vi "IV(H)_DC_vector_magnetsweep_BF_LD-400_K6221_K2182A_PK.vi"() -> ()   [LabVIEW 2016]
uses:
  LabView_Switching exp/SubVI/Keithley 622x LV 8.0/Keithley 622x.lvlib
panel:
  in  "Set Compliance voltage (V)":dbl=2.0 min=0.0 step=0.1 format="%_3f"
  in  "Step 3":dbl[](array[numeric])=[1e-07, 1e-07, 1e-07, 1e-07, 1e-07] min=-3000.0 max=3000.0 format="%.1e"
  in  "To 3":dbl[](array[numeric])=[2e-05, -2e-05, 2e-05, -2e-05, 0.0] min=-3000.0 max=3000.0 format="%.1e"
  in  "From 3":dbl[](array[numeric])=[0.0, 2e-05, -2e-05, 2e-05, -2e-05] min=-3000.0 max=3000.0 format="%.1e"
  in  "wait (ms)":u32=1000
  in  "Nanovoltmeter 2182a VISA":refnum<visa-resource-name>="GPIB0::4::INSTR"
  in  "Current source K6221 VISA":refnum<visa-resource-name>="GPIB0::12::INSTR"
  in  "Number Averaging":i32=50
  in  "Tab Control":enum32{"Page 1", "Page 2"}(tab)
  out "V vs I":cluster{dbl, "Field Reading":dbl}[](graph)=[{88.00020049365409, "Field Reading"=1178949.0151954973}, {88.04984142978704, "Field Reading"=1177290.5042515406}, {88.09983377178898, "Field Reading"=1169991.8797237715}, {88.14983820874596, "Field Reading"=1131113.310921174}, {88.1998015211176, "Field Reading"=1135549.0095311047}, {88.24974082906098, "Field Reading"=1140239.9000253335}, {88.29974217872491, "Field Reading"=1145253.1684029822}, {88.34980121180439, "Field Reading"=1125822.473165846}, {88.39976089537811, "Field Reading"=1100990.7144727584}, {88.44976462735649, "Field Reading"=1124277.980977591}, {88.49991354243424, "Field Reading"=1113133.7403579995}, {88.549835629691, "Field Reading"=1095078.3421750271}, {88.59973785169807, "Field Reading"=1089005.9296407204}, {88.64981796279662, "Field Reading"=1071016.6334025378}, {88.69999071622563, "Field Reading"=1068470.5118392052}, {88.74987372198214, "Field Reading"=1063537.6502689242}, {88.79982875283143, "Field Reading"=1037928.4122448568}, {88.84986306680204, "Field Reading"=1023763.2014216684}, {88.89976547995889, "Field Reading"=1020228.703507441}, {88.94984930717325, "Field Reading"=1000335.3237807469}, {88.99981793410211, "Field Reading"=965050.429505623}, {89.04974778345694, "Field Reading"=978646.5702332633}, {89.09972081248361, "Field Reading"=961519.051741358}, {89.14993565961254, "Field Reading"=939591.945473506}, {89.199725161219, "Field Reading"=918130.4335429888}, {89.24992589877172, "Field Reading"=906781.4220801867}, {89.29974686814681, "Field Reading"=861156.5000297616}, {89.34974265040302, "Field Reading"=831340.4861009503}, {89.39976422439847, "Field Reading"=827959.2552652409}, {89.44974554488792, "Field Reading"=794041.0257164304}, {89.49998047914683, "Field Reading"=792136.3577627148}, {89.54988391763179, "Field Reading"=826457.2883509871}, {89.59982657379398, "Field Reading"=877464.375741542}, {89.64995889945494, "Field Reading"=903593.98825095}, {89.69977125493678, "Field Reading"=917153.966335848}, {89.75002893453679, "Field Reading"=947464.6903531018}, {89.79975720608076, "Field Reading"=968432.2031485286}, {89.84972844020538, "Field Reading"=977841.59734809}, {89.89977155512094, "Field Reading"=992923.8733686475}, {89.9498829635706, "Field Reading"=1004882.2444193498}, {89.99973795869549, "Field Reading"=1028335.1131184339}, {90.04983989122205, "Field Reading"=1025131.272606909}, {90.09994908920751, "Field Reading"=1041173.1024543894}, {90.14982036437434, "Field Reading"=1059237.6751508159}, {90.19980108193258, "Field Reading"=1067565.6836621398}, {90.24973246359373, "Field Reading"=1080472.0318337064}, {90.29996005213907, "Field Reading"=1088475.3372523}, {90.34983233834966, "Field Reading"=1097983.7020025607}, {90.39974610255554, "Field Reading"=1110923.2678247455}, {90.44980343772909, "Field Reading"=1137279.5384549182}, {90.49985241598829, "Field Reading"=1133355.3807623477}, {90.54979294346053, "Field Reading"=1161334.2887808664}, {90.59979410780464, "Field Reading"=1162461.6397829298}, {90.64974434482343, "Field Reading"=1154218.0501570704}, {90.69986742044274, "Field Reading"=1175023.037400592}, {90.74975392715889, "Field Reading"=1158309.8392327735}, {90.80003104609368, "Field Reading"=1160751.9247400747}, {90.84999133832466, "Field Reading"=1180373.5089674825}, {90.89971363302666, "Field Reading"=1178207.0893623114}, {90.9498700750375, "Field Reading"=1186215.801522418}, {90.99972893957116, "Field Reading"=1201413.7681875122}, {91.04977648059084, "Field Reading"=1208681.2076781155}, {91.09985585712178, "Field Reading"=1197895.0972802779}, {91.14982332628642, "Field Reading"=1210652.407715155}, {91.19971838168068, "Field Reading"=1230701.8068384205}, {91.24976729118956, "Field Reading"=1223512.0994189004}, {91.2998516329973, "Field Reading"=1211497.4848096254}, {91.35001158581667, "Field Reading"=1236879.1492508247}, {91.39973785948087, "Field Reading"=1225471.6410425988}, {91.44993058632726, "Field Reading"=1213253.058893187}, {91.49972258715553, "Field Reading"=1210915.25397176}, {91.54988360100296, "Field Reading"=1209863.3661352952}, {91.60003041097399, "Field Reading"=1221964.611924381}, {91.64973262548213, "Field Reading"=1219022.0454230926}, {91.69978400884942, "Field Reading"=1235046.803652391}, {91.74994445658069, "Field Reading"=1232760.0066260807}, {91.80022524347947, "Field Reading"=1256153.8474325093}, {91.8497947448095, "Field Reading"=1241071.9759753507}, {91.89977761295827, "Field Reading"=1249134.9364484414}, {91.94975866856626, "Field Reading"=1235919.8359682774}, {91.99996795172356, "Field Reading"=1235542.8724599753}]
  out "V vs time":cluster{dbl, "Field Reading":dbl}[](graph)=[{1.9999967297364587, "Field Reading"=1178949.0151954973}, {1.999994153904603, "Field Reading"=1177290.5042515406}, {1.9999989129086975, "Field Reading"=1169991.8797237715}, {1.9999918946491422, "Field Reading"=1131113.310921174}, {2.0000099968351024, "Field Reading"=1135549.0095311047}, {1.9999924050786144, "Field Reading"=1140239.9000253335}, {2.0000036443721094, "Field Reading"=1145253.1684029822}, {1.9999972262759285, "Field Reading"=1125822.473165846}, {2.000007931072924, "Field Reading"=1100990.7144727584}, {2.0000066284007425, "Field Reading"=1124277.980977591}, {1.9999952434214299, "Field Reading"=1113133.7403579995}, {1.999996661070107, "Field Reading"=1095078.3421750271}, {2.000006659018672, "Field Reading"=1089005.9296407204}, {2.0000039383733044, "Field Reading"=1071016.6334025378}, {2.0000048869646743, "Field Reading"=1068470.5118392052}, {2.000005777378757, "Field Reading"=1063537.6502689242}, {2.0000049123234382, "Field Reading"=1037928.4122448568}, {1.9999948449122227, "Field Reading"=1023763.2014216684}, {1.9999942408675742, "Field Reading"=1020228.703507441}, {1.999997049209919, "Field Reading"=1000335.3237807469}, {1.9999992434973093, "Field Reading"=965050.429505623}, {2.0000055966816648, "Field Reading"=978646.5702332633}, {1.99999211416235, "Field Reading"=961519.051741358}, {1.999997937140985, "Field Reading"=939591.945473506}, {1.9999920221749543, "Field Reading"=918130.4335429888}, {2.0000099655654218, "Field Reading"=906781.4220801867}, {1.9999941922138977, "Field Reading"=861156.5000297616}, {2.000001391498262, "Field Reading"=831340.4861009503}, {2.000008695947139, "Field Reading"=827959.2552652409}, {1.9999970142052288, "Field Reading"=794041.0257164304}, {2.000004081973531, "Field Reading"=792136.3577627148}, {1.999992656312225, "Field Reading"=826457.2883509871}, {2.0000052739895784, "Field Reading"=877464.375741542}, {2.0000002562870884, "Field Reading"=903593.98825095}, {2.000001858354245, "Field Reading"=917153.966335848}, {1.9999982641352978, "Field Reading"=947464.6903531018}, {1.9999988882792294, "Field Reading"=968432.2031485286}, {2.0000003937283735, "Field Reading"=977841.59734809}, {2.000000600107891, "Field Reading"=992923.8733686475}, {2.000000719113082, "Field Reading"=1004882.2444193498}, {2.000007198020917, "Field Reading"=1028335.1131184339}, {1.9999974916731693, "Field Reading"=1025131.272606909}, {2.0000048080798685, "Field Reading"=1041173.1024543894}, {1.9999906954500268, "Field Reading"=1059237.6751508159}, {1.9999915914078321, "Field Reading"=1067565.6836621398}, {2.0000082879110646, "Field Reading"=1080472.0318337064}, {1.9999953701409292, "Field Reading"=1088475.3372523}, {1.9999996077684985, "Field Reading"=1097983.7020025607}, {2.0000055728717165, "Field Reading"=1110923.2678247455}, {1.9999980037725664, "Field Reading"=1137279.5384549182}, {1.999996384784627, "Field Reading"=1133355.3807623477}, {2.000004103884631, "Field Reading"=1161334.2887808664}, {1.999993443662003, "Field Reading"=1162461.6397829298}, {2.0000021944025916, "Field Reading"=1154218.0501570704}, {1.99999483275991, "Field Reading"=1175023.037400592}, {1.999992715812885, "Field Reading"=1158309.8392327735}, {2.000008000892638, "Field Reading"=1160751.9247400747}, {2.0000043390415403, "Field Reading"=1180373.5089674825}, {2.000008103048867, "Field Reading"=1178207.0893623114}, {1.999990483426892, "Field Reading"=1186215.801522418}, {1.9999901120733596, "Field Reading"=1201413.7681875122}, {1.9999899676610864, "Field Reading"=1208681.2076781155}, {2.000002438619714, "Field Reading"=1197895.0972802779}, {1.99999522928944, "Field Reading"=1210652.407715155}, {2.0000031718988076, "Field Reading"=1230701.8068384205}, {1.9999936301375478, "Field Reading"=1223512.0994189004}, {2.0000077808662033, "Field Reading"=1211497.4848096254}, {2.000008829542967, "Field Reading"=1236879.1492508247}, {2.0000094317080235, "Field Reading"=1225471.6410425988}, {1.9999968576261167, "Field Reading"=1213253.058893187}, {2.000006785911426, "Field Reading"=1210915.25397176}, {1.9999948229255613, "Field Reading"=1209863.3661352952}, {2.000000480747043, "Field Reading"=1221964.611924381}, {2.0000096398922595, "Field Reading"=1219022.0454230926}, {2.0000067770884993, "Field Reading"=1235046.803652391}, {1.9999916662317956, "Field Reading"=1232760.0066260807}, {1.9999971428402814, "Field Reading"=1256153.8474325093}, {1.9999922852387555, "Field Reading"=1241071.9759753507}, {1.9999900072628842, "Field Reading"=1249134.9364484414}, {2.000006765222829, "Field Reading"=1235919.8359682774}, {2.0000011636290265, "Field Reading"=1235542.8724599753}]
  out "Magnetic Field Vector Angle":dbl=91.99996795172356 format="%#_13g"
  out "Magnetic Field Vector magnitude (T)":dbl=2.0000011636290265 format="%#_13g"
  in  "From 2":dbl[](array[numeric])=[2.0] min=-3000.0 max=3000.0 format="%.1g"
  in  "To 2":dbl[](array[numeric])=[2.0] min=-3000.0 max=3000.0 format="%.1g"
  in  "Step 2":dbl[](array[numeric])=[0.5] min=-3000.0 max=3000.0 format="%.3g"
  in  "Wait time after each sweep(min)":dbl=10.0 format="%#_13g"
  out "Z-axis Magnetic Field (T)":string="1.998782856\r\n"
  in  "Y-axis Field ramp rate (T/min)":string="0.01"
  in  "Z-axis Field ramp rate (T/min)":string="0.05"
  out "Z-axis":dbl(slide)=1.998782856 scale=0.0..3.0
  out "Y-Axis":dbl(slide)=-0.069797916 scale=0.0..3.0
  out "Y-axis Magnetic Field (T)":string="-0.069797916\r\n"
  in  "Magnet IP Address Z-axis":string="169.254.239.127"
  in  "Magnet IP Address Y-axis":string="169.254.109.232"
  out "Resistance (ohm)":dbl=1235542.8724599753 format="%#_13g"
  out "Time (s)":dbl=3083.965 format="%#_13g"
  in  "Magnetic field stabilization time (s)":dbl=10.0 format="%#_13g"
  in  "Step":dbl[](array[numeric])=[0.05] min=-3000.0 max=3000.0 format="%.3g"
  in  "To":dbl[](array[numeric])=[92.0] min=-3000.0 max=3000.0 format="%.1f"
  in  "From":dbl[](array[numeric])=[88.0] min=-3000.0 max=3000.0 format="%.1f"
  out "Iset (A)":dbl=3.2552506860087776e-11
  out "Vmeas (V)":dbl=4.02200178316859e-05
  in  "Folder":path=path "D:/Pranava/Data/STS/MA2158 new mask"
  out "data":dbl[](array[numeric])=[2.0000011636290265, 91.99996795172356, 4.02200178316859e-05, 3.2552506860087776e-11, 1235542.8724599753, 3083.965]
  in  "File name":string="009_MA2158[Dev90]_R(A)_baseT_stable_2T_vector_40uV_50ave"
  out "File path":path=path "D:/Pranava/Data/STS/MA2158 new mask/009_MA2158[Dev90]_R(A)_baseT_stable_2T_vector_40uV_50ave.dat"
  # "Z-Axis: In-plane (90 deg)\nY-axis: Out-of-plane (0 deg)"
  # "[Must be less than 0.05]"
  # ".dat"
  # "It is important that there is enough time for the magnet to cool down after each sweep (Typically 15-20 min)"
  # "Configure Field magnitude (T)"
  # "Configure Field Angle (deg)"
  # "Configure current sweeps (A)"
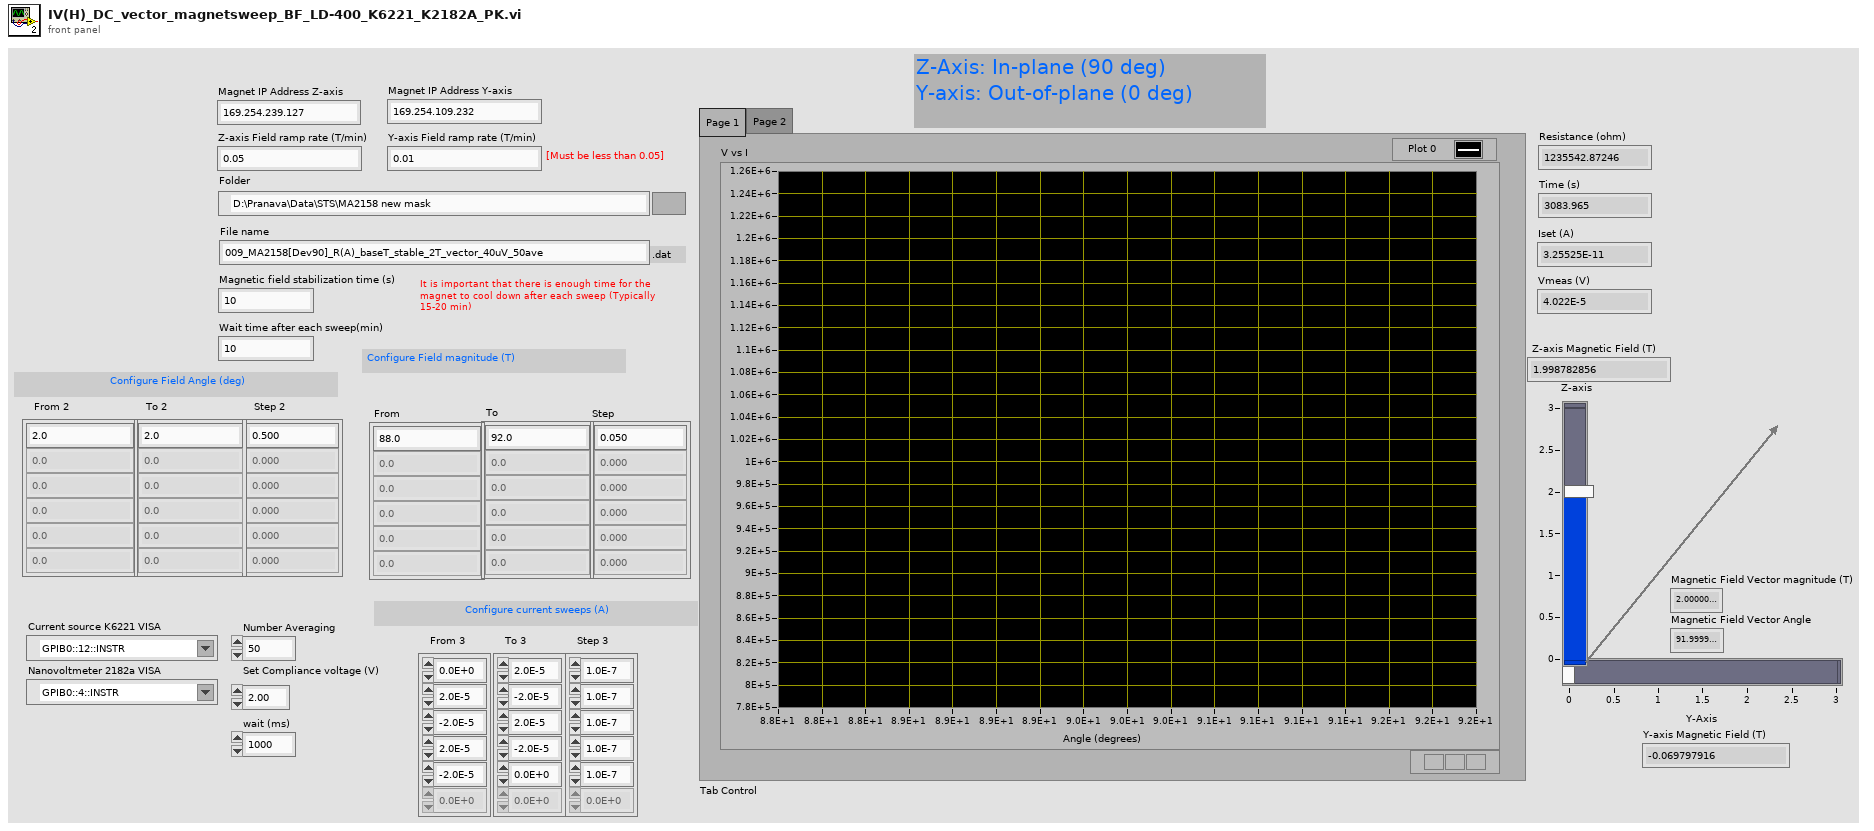
[diagram p1: front panel]
types:
  T1 = enum16{"open", "replace", "create", "open or create", "replace or create", "replace or create with confirmation"}
  T2 = typedef "Keithley 622x.lvlib/KE622x -- Current Level.ctl" = dbl
  T3 = cluster{"Current Level (A)":T2, "Field Reading":dbl}[]
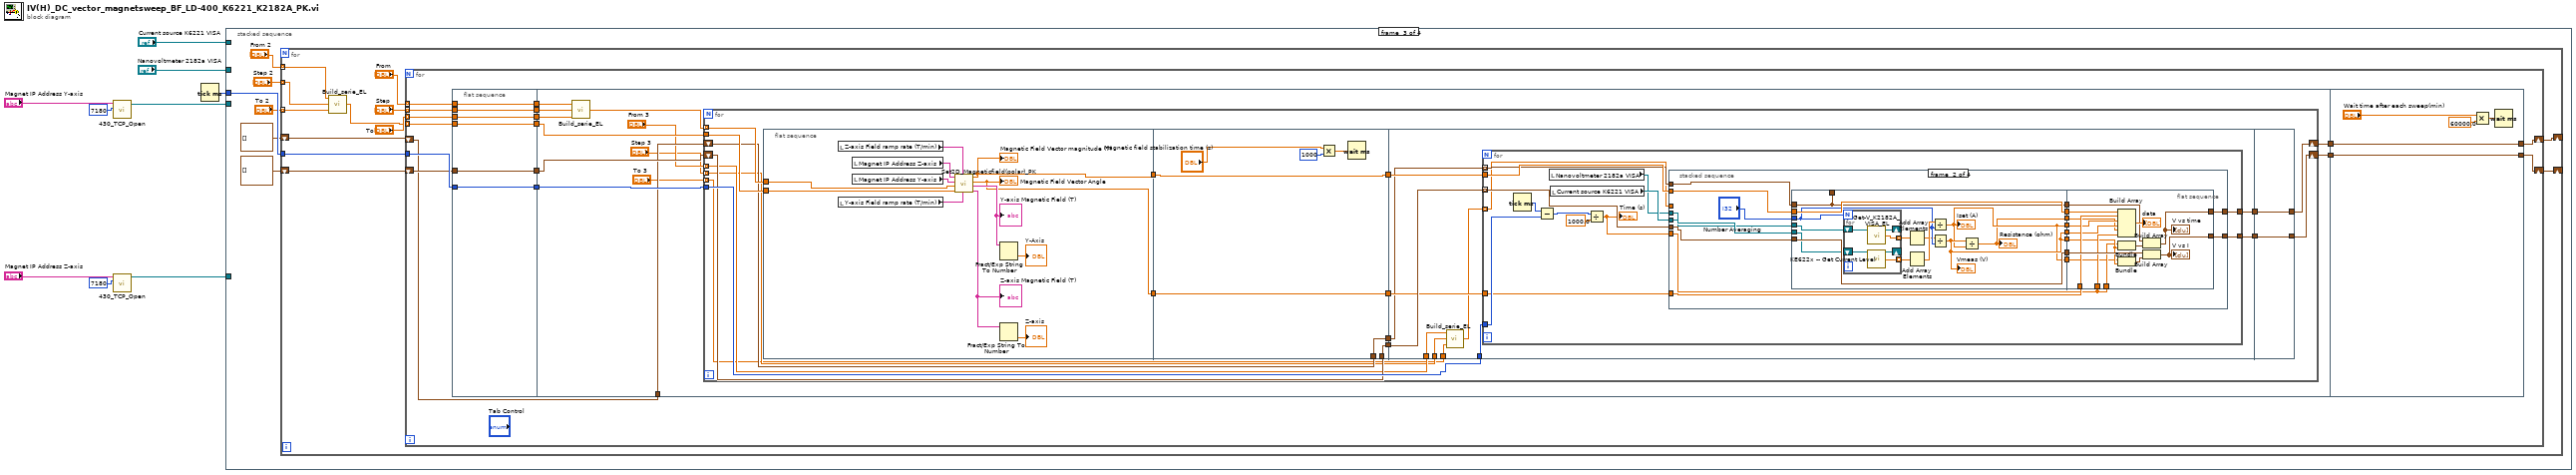
[diagram p0: block diagram]
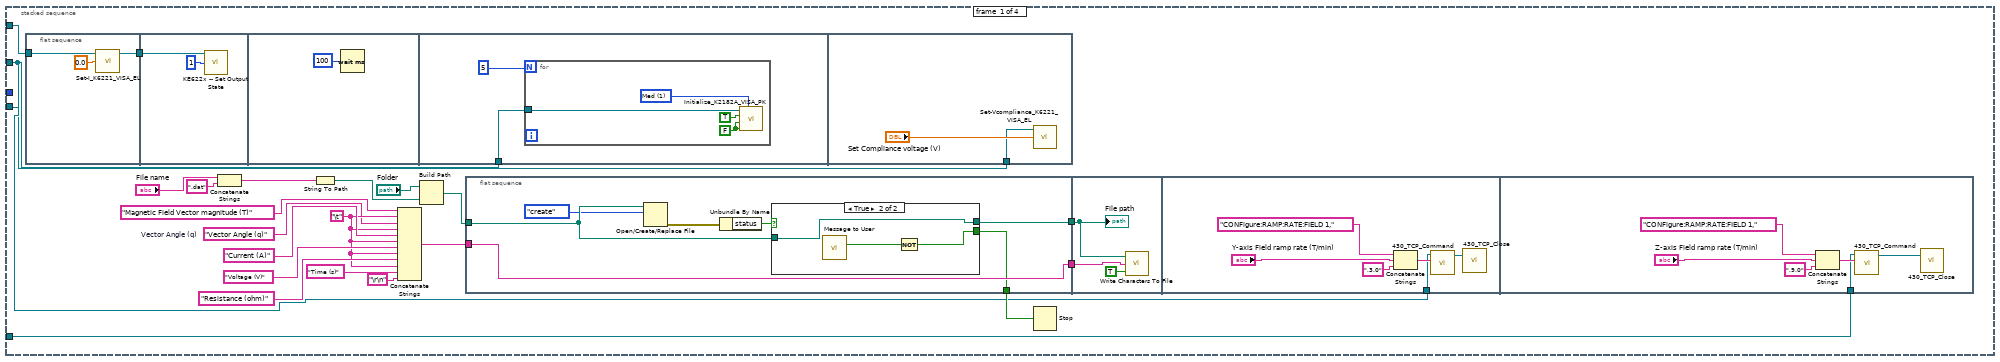
[diagram p2: hidden frame]
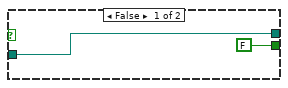
[diagram p3: hidden frame]
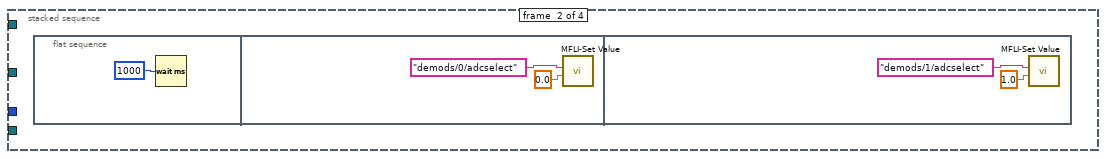
[diagram p4: hidden frame]
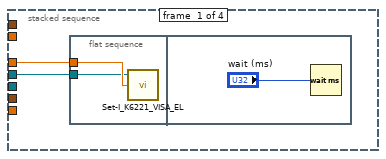
[diagram p5: hidden frame]
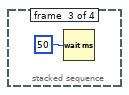
[diagram p6: hidden frame]
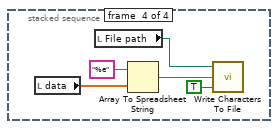
[diagram p7: hidden frame]
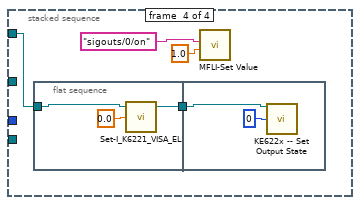
[diagram p8: hidden frame]
diagram:
  n1 = call "430_TCP_Open.vi"("IP Address"="Magnet IP Address Y-axis", "TCP Port"=7180) -> ("connection ID"=w8:refnum<k5>)  [unwired: 4 in, 2 out]
  n2 = call "430_TCP_Open.vi"("IP Address"="Magnet IP Address Z-axis", "TCP Port"=7180) -> ("connection ID"=w3:refnum<k5>)  [unwired: 4 in, 2 out]
  n3 = Tick Count (ms)() -> (millisecond timer value=w7:u32)
  n4 = stacked-sequence {
    tunnel: w8 -> [w18 _ _ _]
    tunnel: w7 -> [_ _ w84 _]
    tunnel: w3 -> [w15 _ _ _]
    tunnel: "Current source K6221 VISA" -> [w11 _ _ w266]
    tunnel: "Nanovoltmeter 2182a VISA" -> [w10 _ _ _]
    frame #0 {
      w13 = "Vector Angle (q)"  # Vector Angle (q)
      w14 = "\t"
      n5 = flat-sequence {
        tunnel: w11 -> [w35]
        tunnel: [w33] -> w12
        tunnel: w12 -> [w37]
        tunnel: w10 -> [w39]
        tunnel: w10 -> [w45]
        frame #0 {
          n6 = call "Set-I_K6221_VISA_EL.vi"("Set I (A)"=0.0, "K6221 VISA"=w35) -> ("K6221 VISA out"=w33:refnum<visa-resource-name>)  [unwired: 2 in, 1 out]
        }
        frame #1 {
          n7 = call "KE622x -- Set Output State.vi"("Resource In"=w37, "Output State"=1) -> ()  [unwired: 12 in, 2 out]
        }
        frame #2 {
          n8 = Wait (ms)(milliseconds to wait=100) -> ()  [unwired: 1 out]
        }
        frame #3 {
          n9 = for {
            N: 5 ("Numeric") -> [_]
            tunnel: w39 -> [w41]
            w43 = u16 1 items=["Slow", "Med", "Fast"] ("Rate (NPLC)")
            w44 = FALSE ("Auto range?")
            n10 = call "Initialize_K2182A_VISA_PK.vi"("VISA address"=w41, "Auto range?"=TRUE, "Analog LPass\nFilter?"=w44, "DC\nFilter?"=w44, "Rate (NPLC)"=w43) -> ()  [unwired: 2 in]
          }
        }
        frame #4 {
          n11 = call "Set-Vcompliance_K6221_VISA_EL.vi"("Set Compliance voltage (V)"="Set Compliance voltage (V)", "K6221 VISA"=w45) -> ()  [unwired: 2 in, 2 out]
        }
      }
      n12 = Concatenate Strings("File name", ".dat" ("string")) -> (w28:string)
      n13 = String To Path(string=w28) -> (path=w20:path)
      n14 = Concatenate Strings("Magnetic Field Vector magnitude (T)", w14, w13, w14, "Current (A)" ("string"), w14, "Voltage (V)" ("string"), w14, "Resistance (ohm)" ("string"), w14, "Time (s)", "\r\n") -> (w29:string)
      n15 = Build Path(base path="Folder", name or relative path=w20) -> (appended path=w19:path)
      n16 = flat-sequence {
        tunnel: w19 -> [w50]
        tunnel: w29 -> [w53]
        tunnel: [w53] -> w32
        tunnel: [w52] -> w26
        tunnel: [w51] -> w31
        tunnel: w32 -> [w60]
        tunnel: w31 -> [w59]
        tunnel: w18 -> [w63]
        tunnel: w15 -> [w68]
        frame #0 {
          n17 = Open/Create/Replace File(file path (use dialog)=w50, operation (0:open)=T1."create") -> (error out=w49:errorcluster)  [unwired: 4 in, 2 out]
          n18 = Unbundle By Name(w49) -> ("status"=w47:bool)
          n19 = case shown="True" w47 {
            tunnel: [FALSE ("Yes") w57] -> w52
            tunnel: [w54 w56] -> w51
            tunnel: w50 -> [w54 w56]
            frame False {
            }
            frame True {
              n20 = call "Message to User"() -> ("Yes"=w58:bool)  [unwired: 10 in, 1 out]
              n21 = Not(x=w58) -> (.not. x?=w57:bool)
            }
          }
        }
        frame #1 {
          n22 = call <vilib>:"Write Characters To File.vi"("append to file? (new file:F)"=TRUE, "character string"=w60, "file path (dialog if empty)"=w59) -> ()  [unwired: 2 in, 1 out]
          "File path" <- w59
        }
        frame #2 {
          n23 = Concatenate Strings("CONFigure:RAMP:RATE:FIELD 1," ("String"), "Y-axis Field ramp rate (T/min)", ",3.0") -> (w64:string)
          n24 = call "430_TCP_Command.vi"("Command"=w64, "connection ID"=w63) -> ("connection ID out"=w67:refnum<k5>)  [unwired: 2 in, 2 out]
          n25 = call "430_TCP_Close.vi"("connection ID"=w67) -> ()  [unwired: 1 in, 2 out]
        }
        frame #3 {
          n26 = Concatenate Strings("CONFigure:RAMP:RATE:FIELD 1," ("String"), "Z-axis Field ramp rate (T/min)", ",9.0") -> (w70:string)
          n27 = call "430_TCP_Command.vi"("Command"=w70, "connection ID"=w68) -> ("connection ID out"=w73:refnum<k5>)  [unwired: 2 in, 2 out]
          n28 = call "430_TCP_Close.vi"("connection ID"=w73) -> ()  [unwired: 1 in, 2 out]
        }
      }
      n29 = Stop(stop? (T)=w26) -> ()
    }
    frame #1 {
      n30 = flat-sequence {
        frame #0 {
          n31 = Wait (ms)(milliseconds to wait=u32 1000) -> ()  [unwired: 1 out]
        }
        frame #1 {
          n32 = call "MFLI-Set Value.vi"("Value"=0.0, "Path"="demods/0/adcselect") -> ()  [unwired: 10 in]
        }
        frame #2 {
          n33 = call "MFLI-Set Value.vi"("Value"=1.0, "Path"="demods/1/adcselect") -> ()  [unwired: 10 in]
        }
      }
    }
    frame #2 {
      n34 = for {
        tunnel: w84 -> [w93]
        shift-right: [w91] -> _
        shift-left: cluster{dbl, "Field Reading":dbl}[] [] -> [w92]
        tunnel: "From 2" -> [w90] mode=indexing
        tunnel: "To 2" -> [w89] mode=indexing
        tunnel: "Step 2" -> [w88] mode=indexing
        shift-right: [w86] -> _
        shift-left: cluster{dbl, "Field Reading":dbl}[] [] -> [w85]
        n35 = call "Build_serie_EL.vi"("end value"=w89, "increment"=w88, "start value"=w90) -> ("output array"=w87:dbl[])
        n36 = for {
          tunnel: "From" -> [w113] mode=indexing
          tunnel: "To" -> [w111] mode=indexing
          tunnel: "Step" -> [w112] mode=indexing
          tunnel: w93 -> [w110]
          shift-right: [w108] -> w91
          shift-left: w92 -> [w109]
          tunnel: w87 -> [w101] mode=indexing
          shift-right: [w99] -> w86
          shift-left: w85 -> [w97]
          n37 = flat-sequence {
            tunnel: w109 -> [w115]
            tunnel: w110 -> [w116]
            tunnel: w111 -> [w117]
            tunnel: w112 -> [w118]
            tunnel: w113 -> [w119]
            tunnel: [w119] -> w107
            tunnel: [w118] -> w106
            tunnel: [w117] -> w105
            tunnel: [w116] -> w104
            tunnel: [w115] -> w103
            tunnel: w101 -> [w114]
            tunnel: [w114] -> w100
            tunnel: w107 -> [w132]
            tunnel: w106 -> [w131]
            tunnel: w105 -> [w130]
            tunnel: w104 -> [w128]
            tunnel: w103 -> [w127]
            tunnel: [w126] -> w102
            tunnel: w100 -> [w125]
            tunnel: [w124] -> w98
            tunnel: w97 -> [w123]
            tunnel: [w265] -> w108
            tunnel: w102 -> [w265]
            tunnel: [w261] -> w99
            tunnel: w98 -> [w261]
            frame #0 {
            }
            frame #1 {
              n38 = call "Build_serie_EL.vi"("end value"=w130, "increment"=w131, "start value"=w132) -> ("output array"=w129:dbl[])
              n39 = for {
                tunnel: w129 -> [w150] mode=indexing
                tunnel: w128 -> [w149]
                shift-right: [w146] -> w126
                shift-left: w127 -> [w147]
                tunnel: w125 -> [w144]
                shift-right: [w138] -> w124
                shift-left: w123 -> [w137]
                tunnel: "From 3" -> [w135] mode=indexing
                tunnel: "Step 3" -> [w134] mode=indexing
                tunnel: "To 3" -> [w133] mode=indexing
                n40 = flat-sequence {
                  tunnel: w150 -> [w151]
                  tunnel: w144 -> [w152]
                  tunnel: [w158] -> w143
                  tunnel: [w153] -> w140
                  tunnel: [w166] -> w148
                  tunnel: w147 -> [w166]
                  tunnel: w143 -> [w165]
                  tunnel: [w165] -> w142
                  tunnel: [w164] -> w141
                  tunnel: w140 -> [w164]
                  tunnel: w137 -> [w163]
                  tunnel: [w163] -> w136
                  tunnel: w149 -> [w180]
                  tunnel: w148 -> [w179]
                  tunnel: [w178] -> w145
                  tunnel: w142 -> [w177]
                  tunnel: w141 -> [w176]
                  tunnel: [w175] -> w139
                  tunnel: w136 -> [w174]
                  tunnel: w135 -> [w172]
                  tunnel: w134 -> [w171]
                  tunnel: w133 -> [w170]
                  tunnel: [w260] -> w146
                  tunnel: w145 -> [w260]
                  tunnel: [w259] -> w138
                  tunnel: w139 -> [w259]
                  frame #0 {
                    n41 = local read "Z-axis Field ramp rate (T/min)"() -> (w159:string)
                    n42 = local read "Y-axis Field ramp rate (T/min)"() -> (w160:string)
                    n43 = local read "Magnet IP Address Z-axis"() -> (w162:string)
                    n44 = local read "Magnet IP Address Y-axis"() -> (w161:string)
                    n45 = call "Set2D_Magneticfield(polar)_PK.vi"("Y-axis Ramp Rate (T/min)"=w160, "Z-axis Ramp Rate (T/min)"=w159, "Set target vector angle (degrees)"=w152, "Set target vector magnitude (T)"=w151, "Y-Axis Magnet IP Address"=w161, "Z-Axis Magnet IP Address"=w162) -> ("Z-axis Magnetic Field (T)"=w155:string, "Y-axis Magnetic Field (T)"=w157:string, "q - Vector angle"=w153:dbl, "R - Vector field magnitude (T)"=w158:dbl)  [unwired: 2 in]
                    "Z-axis Magnetic Field (T)" <- w155
                    "Y-axis Magnetic Field (T)" <- w157
                    "Magnetic Field Vector magnitude (T)" <- w158
                    "Magnetic Field Vector Angle" <- w153
                    n46 = Fract/Exp String To Number(string=w157) -> (number=→"Y-Axis":dbl)  [unwired: 3 in, 1 out]
                    n47 = Fract/Exp String To Number(string=w155) -> (number=→"Z-axis":dbl)  [unwired: 3 in, 1 out]
                  }
                  frame #1 {
                    n48 = Multiply(x="Magnetic field stabilization time (s)", y=1000) -> (x*y=w168:dbl)
                    n49 = Wait (ms)(milliseconds to wait=w168) -> ()  [unwired: 1 out]
                  }
                  frame #2 {
                    n50 = call "Build_serie_EL.vi"("end value"=w170, "increment"=w171, "start value"=w172) -> ("output array"=w173:dbl[])
                    n51 = for {
                      tunnel: w180 -> [w194]
                      tunnel: w179 -> [w193] mode=indexing
                      tunnel: [w192] -> w178
                      tunnel: w177 -> [w187]
                      tunnel: w176 -> [w186]
                      tunnel: [w185] -> w175
                      tunnel: w174 -> [w184] mode=indexing
                      tunnel: w173 -> [w183] mode=indexing
                      n52 = Tick Count (ms)() -> (millisecond timer value=w189:u32)
                      n53 = Subtract(x=w189, y=w194) -> (x-y=w191:u32)
                      n54 = local read "Nanovoltmeter 2182a VISA"() -> (w181:refnum<visa-resource-name>)
                      n55 = local read "Current source K6221 VISA"() -> (w182:refnum<visa-resource-name>)
                      n56 = Divide(x=w191, y=1000.0) -> (x/y=w188:dbl)
                      "Time (s)" <- w188
                      n57 = stacked-sequence {
                        tunnel: w193 -> [_ w216 _ _]
                        tunnel: [_ w217 _ _] -> w192
                        tunnel: w188 -> [_ w202 _ _]
                        tunnel: w187 -> [_ w211 _ _]
                        tunnel: w186 -> [_ w210 _ _]
                        tunnel: [_ w209 _ _] -> w185
                        tunnel: w184 -> [_ w207 _ _]
                        tunnel: w183 -> [w196 _ _ _]
                        tunnel: w182 -> [_ w205 _ _]
                        tunnel: w181 -> [w195 w204 _ _]
                        frame #0 {
                          n58 = flat-sequence {
                            tunnel: w196 -> [w198]
                            tunnel: w195 -> [w197]
                            frame #0 {
                              n59 = call "Set-I_K6221_VISA_EL.vi"("Set I (A)"=w198, "K6221 VISA"=w197) -> ()  [unwired: 2 in, 2 out]
                            }
                            frame #1 {
                              n60 = Wait (ms)(milliseconds to wait="wait (ms)") -> ()  [unwired: 1 out]
                            }
                          }
                        }
                        frame #1 {
                          n61 = flat-sequence {
                            tunnel: [w220] -> w215
                            tunnel: [w230] -> w214
                            tunnel: [w219] -> w213
                            tunnel: [w229] -> w212
                            tunnel: [w228] -> w208
                            tunnel: "Number Averaging" -> [w226]
                            tunnel: w207 -> [w228]
                            tunnel: [w228] -> _
                            tunnel: w216 -> [w230]
                            tunnel: w211 -> [w229]
                            tunnel: w205 -> [w222]
                            tunnel: w204 -> [w221]
                            tunnel: [w220] -> w203
                            tunnel: [w219] -> w201
                            tunnel: [w218] -> w200
                            tunnel: w215 -> [w241]
                            tunnel: [w251] -> w217
                            tunnel: w214 -> [w250]
                            tunnel: w213 -> [w240]
                            tunnel: w212 -> [w245]
                            tunnel: w202 -> [w248]
                            tunnel: w210 -> [w247]
                            tunnel: [w243] -> w209
                            tunnel: w208 -> [w242]
                            tunnel: w203 -> [w244]
                            tunnel: w202 -> [w239]
                            tunnel: w201 -> [w238]
                            tunnel: w200 -> [w237]
                            frame #0 {
                              n62 = for {
                                N: w226 -> [_]
                                tunnel: [w236] -> w225 mode=indexing
                                shift-right: [w232] -> _
                                shift-left: w221 -> [w233]
                                tunnel: [w235] -> w223 mode=indexing
                                shift-right: [w231] -> _
                                shift-left: w222 -> [w234]
                                n63 = call "Get-V_K2182A_VISA_EL.vi"("VISA K2182A"=w233) -> ("V (V)"=w236:dbl, "VISA K2182A out"=w232:refnum<visa-resource-name>)  [unwired: 2 in, 1 out]
                                n64 = call "KE622x -- Get Current Level.vi"("Resource In"=w234) -> ("Resource Out (dupl)"=w231:refnum<visa-resource-name>, "Current Level (A)"=w235:T2)  [unwired: 12 in, 1 out]
                              }
                              n65 = Add Array Elements(numeric array=w225) -> (sum=w224:dbl)
                              n66 = Add Array Elements(numeric array=w223) -> (sum=w227:T2)
                              n67 = Divide(x=w227, y=w226) -> (x/y=w219:T2)
                              "Iset (A)" <- w219
                              n68 = Divide(x=w224, y=w226) -> (x/y=w220:dbl)
                              "Vmeas (V)" <- w220
                              n69 = Divide(x=w220, y=w219) -> (x/y=w218:T2)
                              "Resistance (ohm)" <- w218
                            }
                            frame #1 {
                              n70 = Build Array(w245, w247, w240, w241, w237, w248) -> (→"data":T2[])
                              n71 = Bundle(w239, w244) -> (w246:cluster{dbl, dbl})  [unwired: 1 in]
                              n72 = Bundle("Current Level (A)"=w238, w244) -> (w249:cluster{"Current Level (A)":T2, dbl})  [unwired: 1 in]
                              n73 = Build Array(w242, w246) -> (w243:cluster{dbl, "Field Reading":dbl}[])
                              "V vs time" <- w243
                              n74 = Build Array(w250, w249) -> (w251:T3)
                              "V vs I" <- w251
                            }
                          }
                        }
                        frame #2 {
                          n75 = Wait (ms)(milliseconds to wait=u32 50) -> ()  [unwired: 1 out]
                        }
                        frame #3 {
                          n76 = local read "data"() -> (w254:dbl[])
                          n77 = local read "File path"() -> (w256:path)
                          n78 = Array To Spreadsheet String(array=w254, 3:"%e" ("format string")) -> (spreadsheet string=w257:string)  [unwired: 1 in]
                          n79 = call <vilib>:"Write Characters To File.vi"("append to file? (new file:F)"=TRUE, "character string"=w257, "file path (dialog if empty)"=w256) -> ()  [unwired: 2 in, 1 out]
                        }
                      }
                    }
                  }
                  frame #3 {
                  }
                }
              }
            }
            frame #2 {
              n80 = Multiply(x="Wait time after each sweep(min)", y=60000.0) -> (x*y=w264:dbl)
              n81 = Wait (ms)(milliseconds to wait=w264) -> ()  [unwired: 1 out]
            }
          }
        }
      }
    }
    frame #3 {
      n82 = flat-sequence {
        tunnel: w266 -> [w272]
        tunnel: [w270] -> w267
        tunnel: w267 -> [w274]
        frame #0 {
          n83 = call "Set-I_K6221_VISA_EL.vi"("Set I (A)"=0.0, "K6221 VISA"=w272) -> ("K6221 VISA out"=w270:refnum<visa-resource-name>)  [unwired: 2 in, 1 out]
        }
        frame #1 {
          n84 = call "KE622x -- Set Output State.vi"("Resource In"=w274, "Output State"=0) -> ()  [unwired: 12 in, 2 out]
        }
      }
      n85 = call "MFLI-Set Value.vi"("Value"=1.0, "Path"="sigouts/0/on") -> ()  [unwired: 10 in]
    }
  }
